vi "ENA_Measure Cap.vi"(0 "Semiconductor Module Context":T3, 1 "Meas Type":T2, 2 "Averaging Count":i32=3, 5 "Pins":string[](array[string])=["RF1", "RF2"], 11 "error in (no error)":errorcluster) -> (4 "Semiconductor Module Context Out":T3, 8 "Marker Measurements":T1 {"Port 3 Capacitance" format="%#_6p"; "Port 2 Capacitance" format="%#_6p"; "Port 1 Capacitance" format="%#_6p"}, 15 "error out":errorcluster)   [LabVIEW 2013]
uses:
  <vilib>/NI_TestStand_SemiconductorModule/NI_TestStand_Semiconductor_Module.lvlibp/PinMap/General/SemiconductorModuleContext.ctl
  Controls/Meas Type.ctl
  Controls/ENA_Marker Measurements.ctl
  Pin Map API/ENA Custom Instrument.lvlib
  <vilib>/NI_TestStand_SemiconductorModule/NI_TestStand_Semiconductor_Module.lvlibp
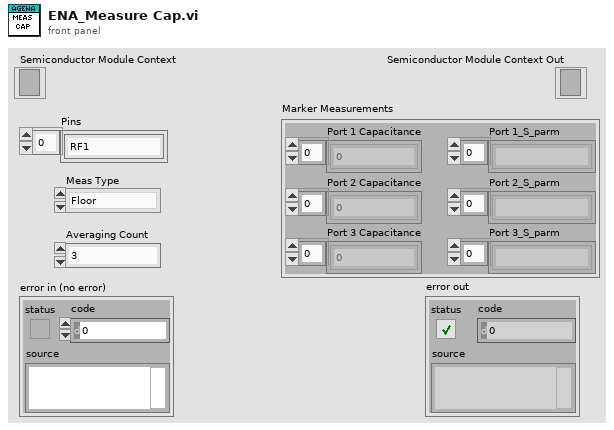
[diagram p1: front panel]
types:
  T1 = typedef "ENA_Marker Measurements.ctl" = cluster{"Port 1 Capacitance":dbl[], "Port 2 Capacitance":dbl[], "Port 3 Capacitance":dbl[], "Port 1_S_parm":string[], "Port 2_S_parm":string[], "Port 3_S_parm":string[]}
  T2 = typedef "Meas Type.ctl" = enum16{"Floor", "Roof", "Buckling", "Charge Transfer"}
  T3 = typedef "NI_TestStand_Semiconductor_Module.lvlibp/SemiconductorModuleContext.ctl" = refnum<k7>
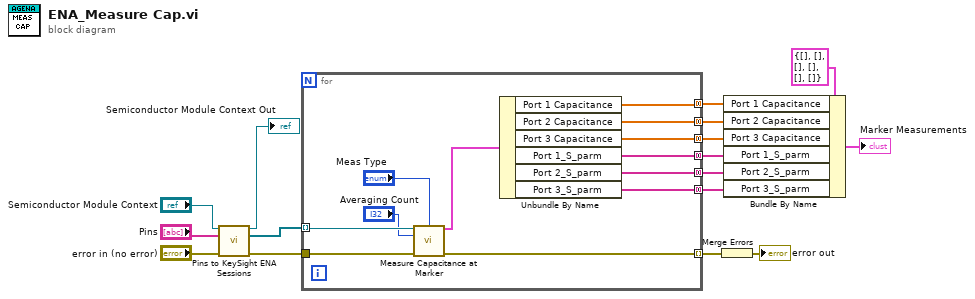
[diagram p0: block diagram]
diagram:
  n1 = call "Pins to KeySight ENA Sessions.vi"("Semiconductor Module Context"="Semiconductor Module Context", "Pins"="Pins", "error in (no error)"="error in (no error)") -> ("Semiconductor Module Context Out"=→"Semiconductor Module Context Out":T3, "Instrument Sessions"=w14:refnum<visa-resource-name>[], "error out"=w15:errorcluster)  [unwired: 8 in, 2 out]
  n2 = for {
    tunnel: w14 -> [w27] mode=indexing
    tunnel: w15 -> [w28]
    tunnel: [w26] -> w9 mode=indexing
    tunnel: [w22] -> w6 mode=concatenating
    tunnel: [w21] -> w5 mode=concatenating
    tunnel: [w20] -> w4 mode=concatenating
    tunnel: [w19] -> w3 mode=concatenating
    tunnel: [w18] -> w2 mode=concatenating
    tunnel: [w17] -> w1 mode=concatenating
    n3 = call "Measure Capacitance at Marker.vi"("VISA resource name"=w27, "Meas Type"="Meas Type", "Averaging Count"="Averaging Count", "Error In"=w28) -> ("Marker Measurements"=w23:T1, "Error Out"=w26:errorcluster)  [unwired: 10 in]
    n4 = Unbundle By Name(w23) -> ("Port 1 Capacitance"=w22:dbl[], "Port 2 Capacitance"=w21:dbl[], "Port 3 Capacitance"=w20:dbl[], "Port 1_S_parm"=w19:string[], "Port 2_S_parm"=w18:string[], "Port 3_S_parm"=w17:string[])
  }
  n5 = Merge Errors(w9) -> (→"error out":errorcluster)
  n6 = Bundle By Name(cluster=T1 {"Port 1 Capacitance"=[], "Port 2 Capacitance"=[], "Port 3 Capacitance"=[], "Port 1_S_parm"=[], "Port 2_S_parm"=[], "Port 3_S_parm"=[]} ("Marker Measurements 2"), "Port 1 Capacitance"=w6, "Port 2 Capacitance"=w5, "Port 3 Capacitance"=w4, "Port 1_S_parm"=w3, "Port 2_S_parm"=w2, "Port 3_S_parm"=w1) -> (→"Marker Measurements":T1)
